vi "liniowy.vi"(1 "ilosc probek":u32=1000, 2 "F min":dbl=100.0, 3 "F max":dbl=100000.0) -> (0 "Tabela":T1[](array[typedef]))   [LabVIEW 2021]
uses:
  controlmaszyna.ctl
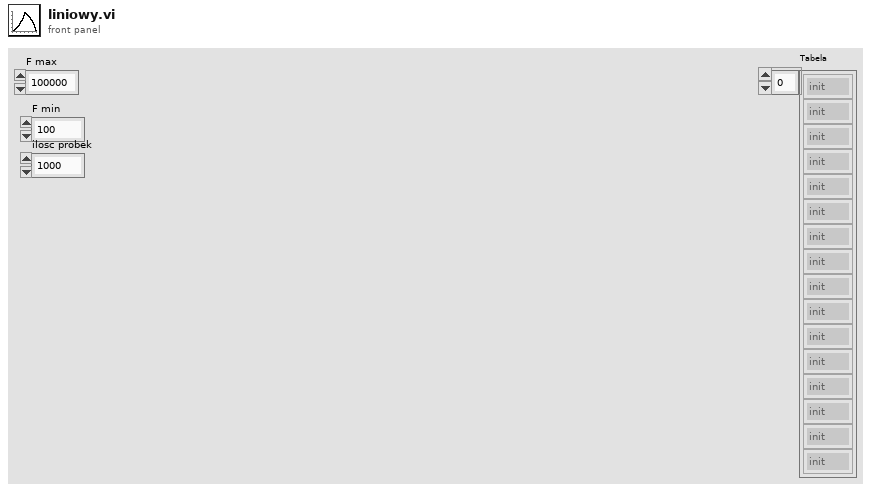
[diagram p1: front panel]
types:
  T1 = typedef "controlmaszyna.ctl" = enum16{"init", "praca", "pomiar", "wykres", "zapis", "stop", "koniec"}
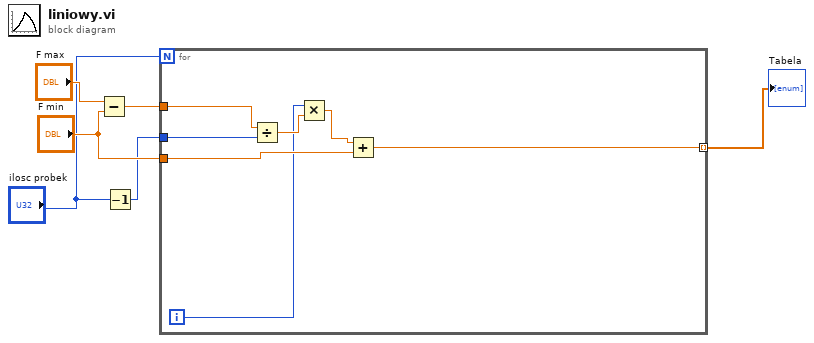
[diagram p0: block diagram]
diagram:
  n1 = Subtract(x="F max", y="F min") -> (x-y=w5:dbl)
  n2 = Decrement(x="ilosc probek") -> (x-1=w1:u32)
  n3 = for {
    N: "ilosc probek" -> [_]
    tunnel: w5 -> [w13]
    tunnel: "F min" -> [w12]
    tunnel: [w8] -> w3 mode=indexing
    tunnel: w1 -> [w7]
    i -> [w9]
    n4 = Divide(x=w13, y=w7) -> (x/y=w10:dbl)
    n5 = Multiply(x=w9, y=w10) -> (x*y=w11:dbl)
    n6 = Add(x=w11, y=w12) -> (x+y=w8:dbl)
  }
  "Tabela" <- w3
